vi "readNbrLinCol (SubVI).vi"(11 "tabIma":u16[][](array[numeric])) -> (2 "nbrCol":i32, 3 "nbrLine":i32)   [LabVIEW 2020, in "Logging.lvlib"]
uses:
  LOGGING/Logging.lvlib
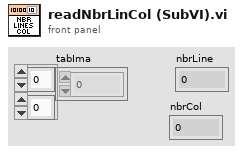
[diagram p1: front panel]
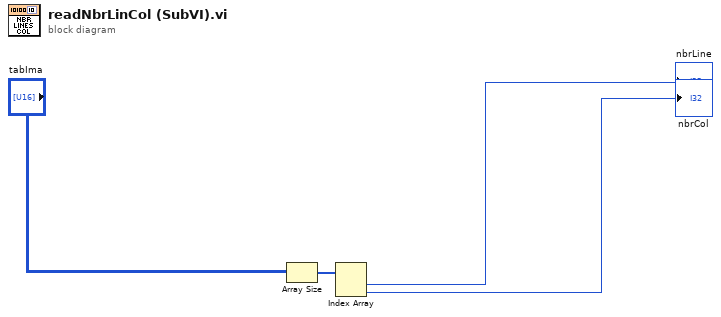
[diagram p0: block diagram]
diagram:
  n1 = Array Size(array="tabIma") -> (size(s)=w1:i32[])
  n2 = Index Array(array=w1) -> (element #1=→"nbrLine":i32, element #2=→"nbrCol":i32)  [unwired: 2 in]
